vi "Login.vi"(0 "reference in":refnum<class "Login_Base.lvclass">, 11 "error in (no error)":errorcluster) -> (4 "reference in":refnum<class "Login_Base.lvclass">, 6 "User":string, 8 "valid":bool, 10 "Rights":string[](array[string]), 13 "Pwd":string, 14 "Cancelled":bool, 15 "error out":errorcluster)   [LabVIEW 2022 SP3, in "Login_Base.lvlib" / "Login_Base.lvclass"]
uses:
  Login_Base.lvclass
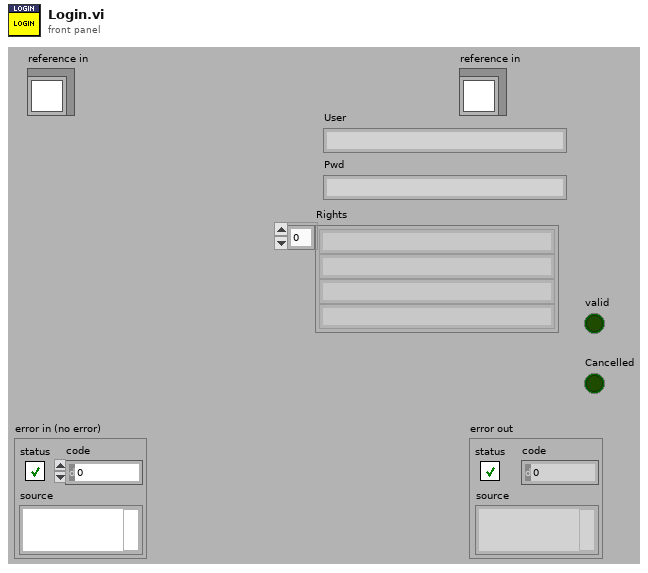
[diagram p1: front panel]
types:
  T1 = typedef "Login_Base.lvlib/Login_Base.lvclass/ObjectAttributes.ctl" = cluster{"Config":T2}
  T2 = typedef "Login_Base.lvlib/Login_Base.lvclass/Config.ctl" = cluster{"default":string}
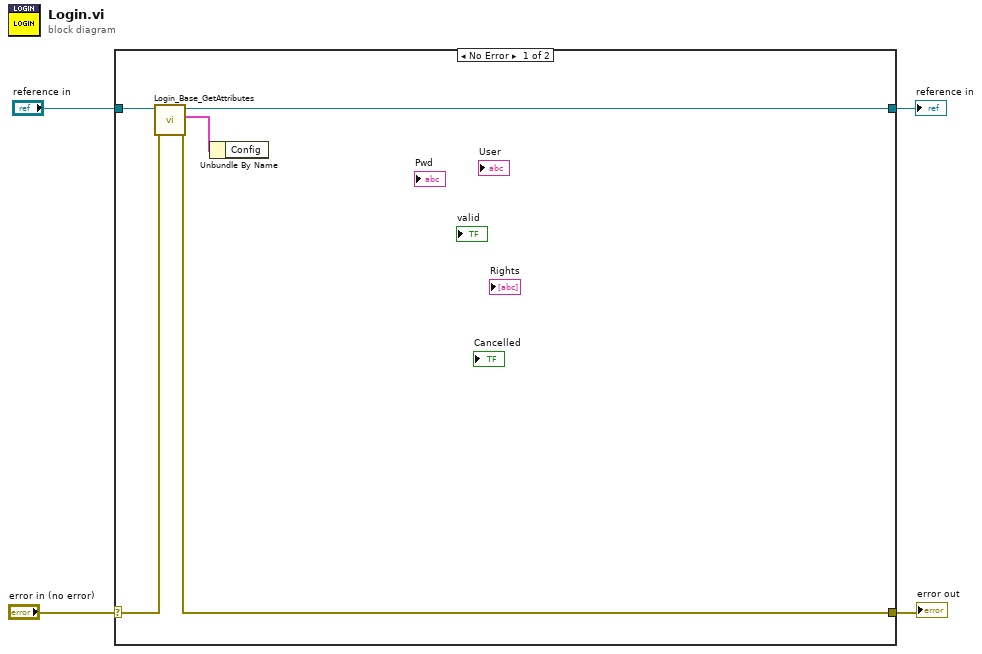
[diagram p0: block diagram]
diagram:
  n1 = case shown="No Error" "error in (no error)" {
    selector: "error in (no error)" -> [w9 w11]
    tunnel: [w7 w11] -> w3
    tunnel: [w5 w10] -> w1
    tunnel: "reference in" -> [w6 w10]
    frame No Error {
      n2 = call "Login_Base_GetAttributes.vi"("error in (no error)"=w9, "reference in"=w6) -> ("error out"=w7:errorcluster, "Data"=w8:T1, "reference out"=w5:refnum<class "Login_Base.lvclass">)  [unwired: 6 in, 1 out]
      n3 = Unbundle By Name(w8) -> ()  [unwired: 1 out]
    }
    frame Error {
    }
  }
  "error out" <- w3
  "reference in" <- w1
